vi "checkout_book.vi"(8 "error in (no error)":errorcluster, 10 "book title":string, 11 "client in":refnum<class "client.lvclass">) -> (0 "error out":errorcluster, 3 "client out":refnum<class "client.lvclass">)   [LabVIEW 2020, in "client.lvclass"]
uses:
  client.lvclass
  client.lvclass/client.ctl
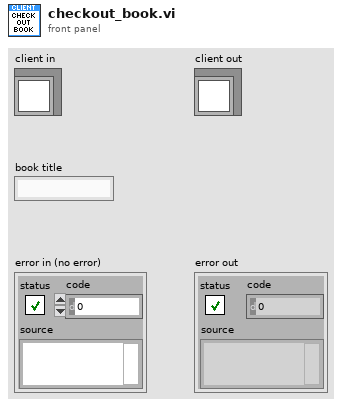
[diagram p1: front panel]
types:
  T1 = cluster{"exit event":refnum<user-event>, "checkout event":refnum<user-event>, "checkin event":refnum<user-event>}
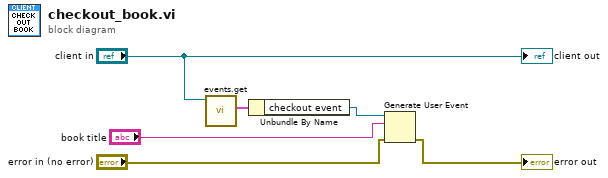
[diagram p0: block diagram]
diagram:
  n1 = call "events.get.vi"("librarian_sm in"="client in") -> ("events"=w2:T1)  [unwired: 9 in, 1 out]
  n2 = Unbundle By Name(w2) -> ("checkout event"=w1:refnum<user-event>)
  n3 = Generate User Event(user event=w1, event data cluster="book title", error in="error in (no error)") -> (error out=→"error out":errorcluster)  [unwired: 1 in, 1 out]
  "client out" <- "client in"
